vi "Get SMO PGSQL Log Paths.vi"(5 "getAll Cluster":variant, 7 "Paths":string="llab_038:d000(TEST_TABLE--Temperature(Kelvin))\nllab_038:d002(TEST_TABLE--voltage 2(volts))\nllab_038:b000(TEST_TABLE--ON?())\nllab_038:v001(TEST_TABLE--sample())", 8 "error in (no error)":errorcluster, 11 "Inst.Attocube-3DR in":refnum<class "Inst.Attocube-3DR.lvclass">) -> (0 "error out":errorcluster, 2 "Paths":string, 3 "Inst.Attocube-3DR out":refnum<class "Inst.Attocube-3DR.lvclass">)   [LabVIEW 2019, in "Inst.Attocube-3DR.lvclass"]
uses:
  Inst.Attocube-3DR.lvclass
  Typedefs/Inst.Attocube-3DR.getAll--Cluster.ctl
  <userlib>/LevyLab/LV-Data/LV-Data.PG/API/Write Variable (one-row).vi
  <userlib>/LevyLab/Instrument Framework/Instrument Types/VSource/Instrument.VSource.lvclass
  <userlib>/LevyLab/LV-Data/LV-Data.PG/LV-Data.PGSQL.lvclass
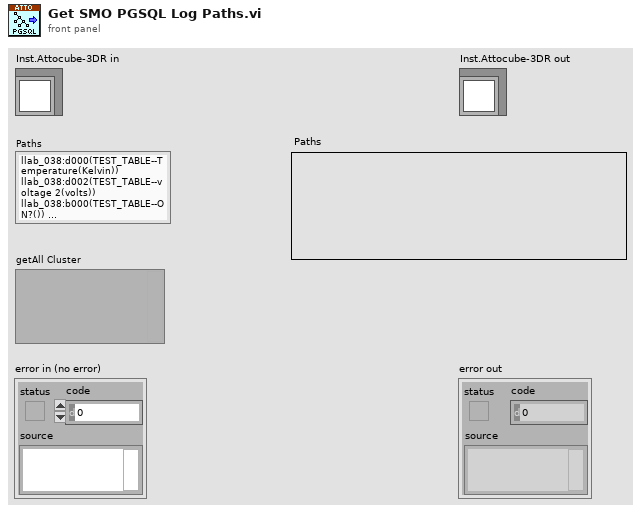
[diagram p1: front panel]
types:
  T1 = typedef "Inst.Attocube-3DR.lvclass/Inst.Attocube-3DR.getAll--Cluster.ctl" = cluster{"Axis 1: Amplitude":i32, "Axis 1: Capacitance":i32, "Axis 1: Current Position":i32, "Axis 1: DCLevel":i32, "Axis 1: Frequency":i32, "Axis 1: StepWidth":i32, "Axis 1: control mode":i32, "Axis 1: rot. count":i32, "Axis 1: sp position":i32, "Axis 1: sp rot. count":i32, "Axis 1: speed":i32, "Axis 1: Target GND":bool, "Axis 1: Output":bool, "Axis 1: Single Circle Mode":bool, "Axis 1: moving":bool, "Axis 1: stop detected":bool, "Axis 1:  sensor error":bool, "Axis 1: sensor diconnected":bool, "Axis 1: stop enable":bool, "Axis 2: Current Position":i32, "Axis 2: DCLevel":i32, "Axis 2: Frequency":i32, "Axis 2: StepWidth":i32, "Axis 2: control mode":i32, "Axis 2: rot. count":i32, "Axis 2: sp position":i32, "Axis 2: sp rot. count":i32, "Axis 2: speed":i32, "Axis 2: Capacitance":i32, "Axis 2: Amplitude":i32, "Axis 2: Target GND":bool, "Axis 2: Output":bool, "Axis 2: Single Circle Mode":bool, "Axis 2: moving":bool, "Axis 2: stop detected":bool, "Axis 2:  sensor error":bool, "Axis 2: sensor diconnected":bool, "Axis 2: stop enable":bool}
  T2 = cluster{"Axis 1: Current Position":i32, "Axis 1: Capacitance":i32, "Axis 1: Amplitude":i32, "Axis 1: Frequency":i32, "Axis 2: Current Position":i32, "Axis 2: Capacitance":i32, "Axis 2: Frequency":i32, "Axis 2: Amplitude":i32}
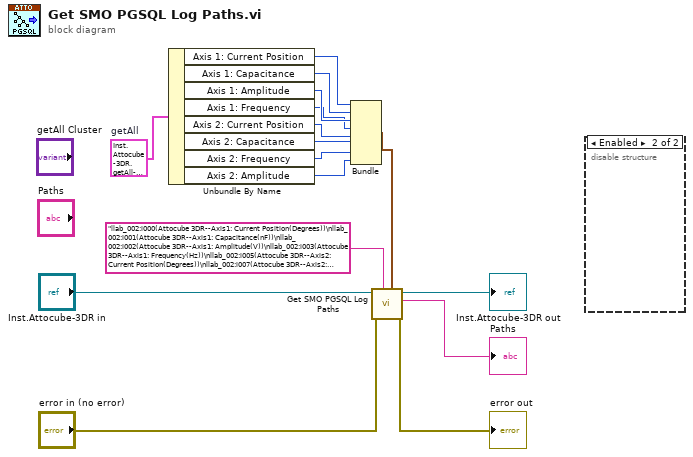
[diagram p0: block diagram]
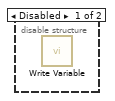
[diagram p2: hidden frame]
diagram:
  w10 = T1 {"Axis 1: Amplitude"=0, "Axis 1: Capacitance"=0, "Axis 1: Current Position"=0, "Axis 1: DCLevel"=0, "Axis 1: Frequency"=0, "Axis 1: StepWidth"=0, "Axis 1: control mode"=0, "Axis 1: rot. count"=0, "Axis 1: sp position"=0, "Axis 1: sp rot. count"=0, "Axis 1: speed"=0, "Axis 1: Target GND"=FALSE, "Axis 1: Output"=FALSE, "Axis 1: Single Circle Mode"=FALSE, "Axis 1: moving"=FALSE, "Axis 1: stop detected"=FALSE, "Axis 1:  sensor error"=FALSE, "Axis 1: sensor diconnected"=FALSE, "Axis 1: stop enable"=FALSE, "Axis 2: Current Position"=0, "Axis 2: DCLevel"=0, "Axis 2: Frequency"=0, "Axis 2: StepWidth"=0, "Axis 2: control mode"=0, "Axis 2: rot. count"=0, "Axis 2: sp position"=0, "Axis 2: sp rot. count"=0, "Axis 2: speed"=0, "Axis 2: Capacitance"=0, "Axis 2: Amplitude"=0, "Axis 2: Target GND"=FALSE, "Axis 2: Output"=FALSE, "Axis 2: Single Circle Mode"=FALSE, "Axis 2: moving"=FALSE, "Axis 2: stop detected"=FALSE, "Axis 2:  sensor error"=FALSE, "Axis 2: sensor diconnected"=FALSE, "Axis 2: stop enable"=FALSE}  # getAll
  n1 = Unbundle By Name(w10) -> ("Axis 1: Current Position"=w8:i32, "Axis 1: Capacitance"=w7:i32, "Axis 1: Amplitude"=w6:i32, "Axis 1: Frequency"=w4:i32, "Axis 2: Current Position"=w5:i32, "Axis 2: Capacitance"=w3:i32, "Axis 2: Frequency"=w2:i32, "Axis 2: Amplitude"=w1:i32)
  n2 = Bundle("Axis 1: Current Position"=w8, "Axis 1: Capacitance"=w7, "Axis 1: Amplitude"=w6, "Axis 1: Frequency"=w4, "Axis 2: Current Position"=w5, "Axis 2: Capacitance"=w3, "Axis 2: Frequency"=w2, "Axis 2: Amplitude"=w1) -> (w9:T2)  [unwired: 1 in]
  n3 = call-parent "Get SMO PGSQL Log Paths.vi"("getAll Cluster"=w9, "Default Paths"="llab_002:i000(Attocube 3DR--Axis1: Current Position(Degrees))\nllab_002:i001(Attocube 3DR--Axis1: Capacitance(nF))\nllab_002:i002(Attocube 3DR--Axis1: Amplitude(V))\nllab_002:i003(Attocube 3DR--Axis1: Frequency(Hz))\nllab_002:i005(Attocube 3DR--Axis2: Current Position(Degrees))\nllab_002:i007(Attocube 3DR--Axis2: Capacitance(nF))\nllab_002:i004(Attocube 3DR--Axis2: Frequency(Hz))\nllab_002:i006(Attocube 3DR--Axis2: Amplitude(V))" ("Paths"), "error in (no error)"="error in (no error)", "Instrument in"="Inst.Attocube-3DR in") -> ("error out"=→"error out":errorcluster, "Paths"=→"Paths":string, "Instrument out"=→"Inst.Attocube-3DR out":refnum<class "Inst.Attocube-3DR.lvclass">)  [unwired: 5 in]
  n4 = disable-structure shown="Enabled" {
    frame Disabled {
      n5 = call-poly <userlib>:"Write Variable.vi"() -> ()  [unwired: 8 in, 4 out]
    }
    frame Enabled {
    }
  }
